vi "zmq_socket_monitor.vi"(4 "error in":errorcluster, 5 "endpoint in":string, 6 "filter (all events)":T1[](array[typedef]), 7 "socket in":refnum<class "zmq_socket.lvclass">) -> (0 "error out":errorcluster, 1 "endpoint out":string, 2 "mask":i32, 3 "socket out":refnum<class "zmq_socket.lvclass">)   [LabVIEW 2019, in "zeromq.lvlib" / "zmq_socket.lvclass"]
doc: "Sets up a socket monitor which checks for events on the input socket, and posts them to the provided endpoint (which should be on the inproc protocol). Only events matching the given type will be passed on.\n\nOnce the monitor has been started, a ZMQ_PAIR socket should be connected to the endpoint and will receive binary information about the events. The zmq_get_monitor_event.vi is provided to decode this information into readable form.\n\nDetailed API documentation: http://api.zeromq.org/3-2:zmq-socket-monitor"
uses:
  zmq_socket.lvclass
  monitor_event.ctl
  zmq_socket.lvclass/zmq_socket.ctl
  <vilib>/Utility/error.llb/Error Cluster From Error Code.vi
  zeromq.lvlib
panel:
  # "ØMQ"
  # "labview"
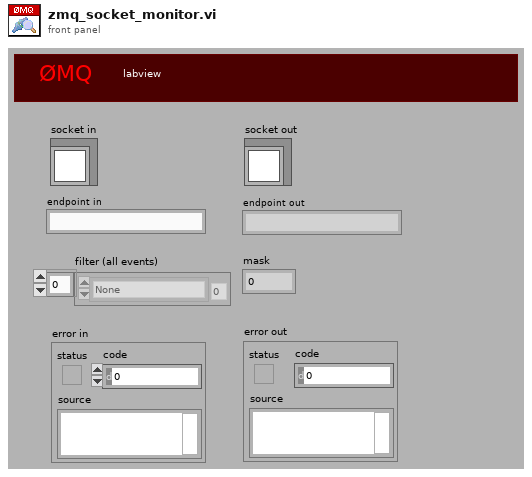
[diagram p1: front panel]
types:
  T1 = typedef "zeromq.lvlib/monitor_event.ctl" = enum8{"None", "Connected", "Connect Delayed", "Connect Retry", "Listening", "Bind Failed", "Accepted", "Accept Failed", "Closed", "Close Failed", "Disconnected"}
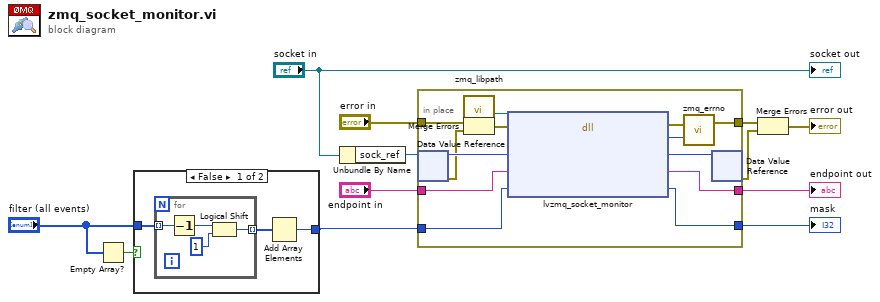
[diagram p0: block diagram]
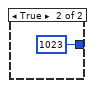
[diagram p2: hidden frame]
diagram:
  n1 = Empty Array?(array="filter (all events)") -> (empty?=w8:bool)
  n2 = case shown="False" w8 {
    tunnel: "filter (all events)" -> [w15 _]
    tunnel: [w13 1023] -> w6
    frame False {
      n3 = for {
        tunnel: w15 -> [w19] mode=indexing
        tunnel: [w16] -> w14 mode=indexing
        n4 = Decrement(x=w19) -> (x-1=w18:T1)
        n5 = Logical Shift(y=w18, x=1) -> (x << y=w16:i32)
      }
      n6 = Add Array Elements(numeric array=w14) -> (sum=w13:i32)
    }
    frame True {
    }
  }
  n7 = Unbundle By Name("socket in") -> ("sock_ref"=w9:refnum<data-value>)
  n8 = in-place {
    in-place-border: "endpoint in" -> [w33]
    in-place-border: "error in" -> [w23]
    in-place-border: [w30] -> w3
    in-place-border: w6 -> [w26]
    in-place-border: [w25] -> w5
    in-place-border: [w24] -> w4
    n9 = in-place-dvr #1(w9) -> (w29:u64, w21:errorcluster)
    n10 = call "zmq_libpath.vi"() -> ("path"=w27:path)
    n11 = Merge Errors(w23, w21) -> (w22:errorcluster)
    n12 = dll-call lib="?" fn="lvzmq_socket_monitor" ("zmq_labview.dll:lvzmq_connect")(path in=w27, error in=w22, "sock_obj"=w29, "endpoint"=w33, "mask"=w26) -> (error out=w32:errorcluster, "return type"=w31:i32, "sock_obj"=w28:u64, "endpoint"=w25:string, "mask"=w24:i32)  [unwired: 1 in, 1 out]
    n13 = call "zmq_errno.vi"("retval"=w31, "error in"=w32) -> ("error out"=w30:errorcluster)  [unwired: 1 out]
    n14 = in-place-dvr #1(w28) -> (w2:errorcluster)  [unwired: 1 out]
  }
  "endpoint out" <- w5
  "mask" <- w4
  n15 = Merge Errors(w3, w2) -> (→"error out":errorcluster)
  "socket out" <- "socket in"
